vi "FPGA_DAC_move.vi"   [LabVIEW 2013]
uses:
  <vilib>/rvi/Emulation/niFpgaSctlEmulationGetInTimedLoop.vi
  <vilib>/rvi/Emulation/niFpgaEmulationReportErrorSimple.vi
  <vilib>/rvi/Emulation/niFpgaGetClockAttributes.vi
  <vilib>/rvi/FIFO/Fifo_Resource/nirvififoEmulationReadFpgaImpl.vi
  <vilib>/rvi/DataTransferAndStorage/Container/Common/niFpgaContainerGetUniqueNameForEmu.vi
  <vilib>/rvi/Emulation/niFpgaCriticalErrorInLSC.vi
  <vilib>/rvi/eio/common/nirviEmuTemplateMethod_errors.vi
  <vilib>/rvi/DataTransferAndStorage/Container/XNode/niFpgaContainer.xnode
  <vilib>/rvi/FIFO/Fifo_Resource/nirvififoEmulationRead.vi
  <vilib>/eio/EIONode/EIONode.xnode
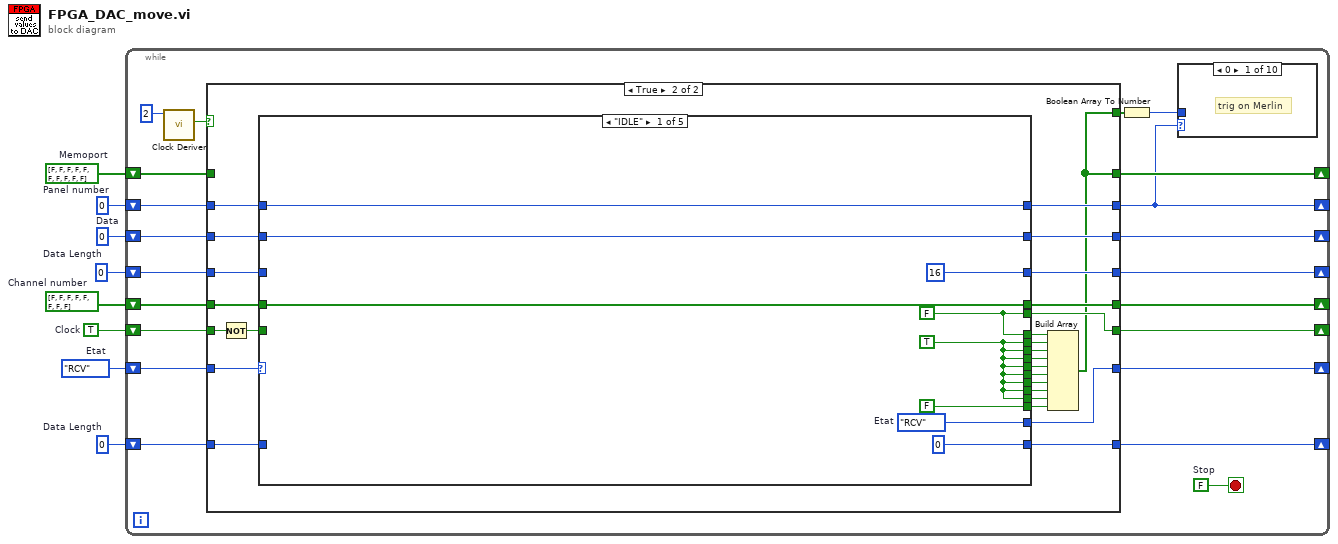
[diagram p0: block diagram]
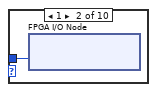
[diagram p2: hidden frame]
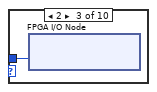
[diagram p3: hidden frame]
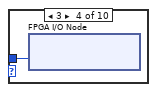
[diagram p4: hidden frame]
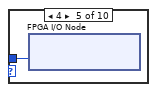
[diagram p5: hidden frame]
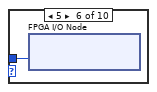
[diagram p6: hidden frame]
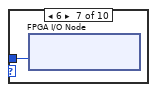
[diagram p7: hidden frame]
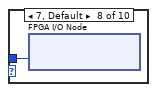
[diagram p8: hidden frame]
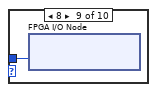
[diagram p9: hidden frame]
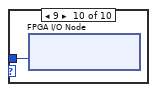
[diagram p10: hidden frame]
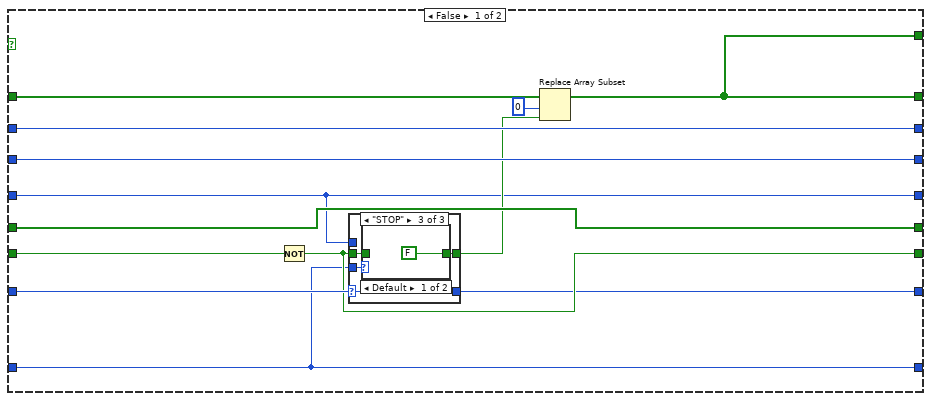
[diagram p11: hidden frame]
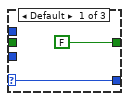
[diagram p12: hidden frame]
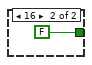
[diagram p14: hidden frame]
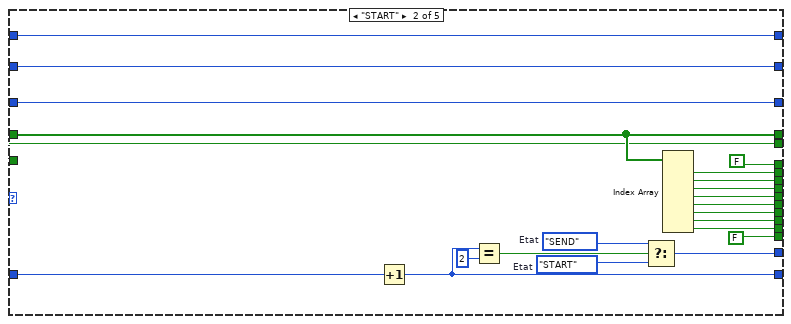
[diagram p16: hidden frame]
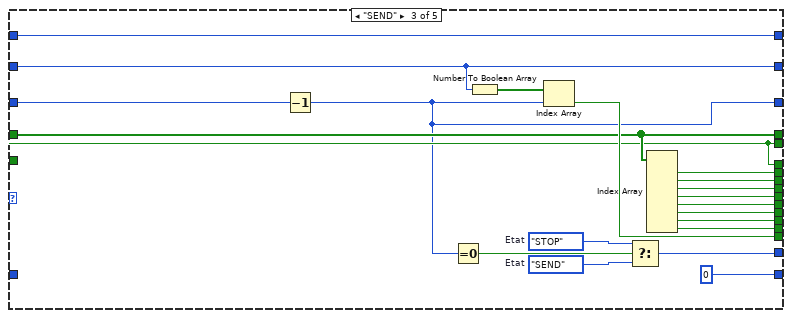
[diagram p17: hidden frame]
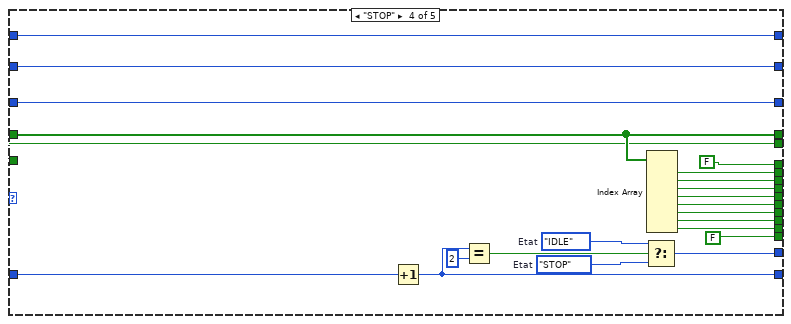
[diagram p18: hidden frame]
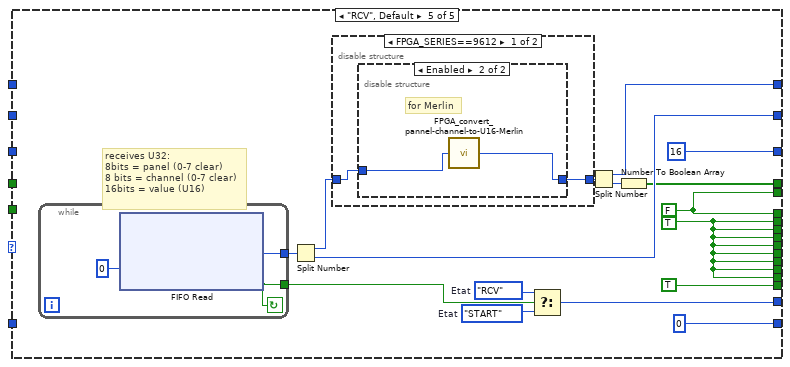
[diagram p19: hidden frame]
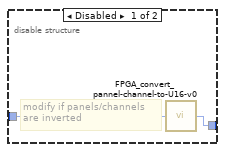
[diagram p20: hidden frame]
diagram:
  w1 = enum8{"IDLE", "START", "SEND", "STOP", "RCV"}."RCV"  # Etat
  w8 = u8 0  # Panel number
  w7 = bool[] [FALSE, FALSE, FALSE, FALSE, FALSE, FALSE, FALSE, FALSE]  # Channel number
  w6 = bool[] [FALSE, FALSE, FALSE, FALSE, FALSE, FALSE, FALSE, FALSE, FALSE, FALSE]  # Memoport
  w5 = u8 0  # Data Length
  w4 = 0  # Data Length
  w3 = u16 0  # Data
  w2 = TRUE  # Clock
  n1 = while {
    shift-right: [w23] -> _
    shift-left: w2 -> [w20]
    shift-right: [w29] -> _
    shift-left: w1 -> [w10]
    shift-right: [w28] -> _
    shift-left: w3 -> [w25]
    shift-right: [w27] -> _
    shift-left: w4 -> [w26]
    shift-right: [w22] -> _
    shift-left: w5 -> [w24]
    shift-right: [w19] -> _
    shift-left: w6 -> [w18]
    shift-right: [w17] -> _
    shift-left: w7 -> [w16]
    shift-right: [w13] -> _
    shift-left: w8 -> [w14]
    stop <- w9 stop-if-true
    w9 = FALSE  # Stop
    n2 = call "Clock Deriver.vi"("Divisor"=u32 2) -> ("Clock Out"=w21:bool)  [unwired: 1 in, 9 out]
    n3 = case shown="True" w21 {
      tunnel: w10 -> [w44 w91]
      tunnel: [w39 w90] -> w29
      tunnel: [w51 w89] -> w28
      tunnel: [w40 w88] -> w27
      tunnel: w26 -> [w40 w87]
      tunnel: w25 -> [w51 w86]
      tunnel: w20 -> [w47 w70]
      tunnel: w24 -> [w41 w85]
      tunnel: [w43 w69] -> w23
      tunnel: [w41 w84] -> w22
      tunnel: [w45 w67] -> w19
      tunnel: w18 -> [w50 _]
      tunnel: [w48 w75] -> w17
      tunnel: w16 -> [w48 w74]
      tunnel: [w46 w72] -> w13
      tunnel: w14 -> [w46 w73]
      tunnel: [w45 w67] -> w11
      frame False {
        n4 = Not(x=w47) -> (.not. x?=w43:bool)
        n5 = case shown="\"STOP\"" w44 {
          selector: w44 -> [w52 w54 w60]
          tunnel: w43 -> [_ w57 w62]
          tunnel: [FALSE w56 w61] -> w42
          tunnel: w41 -> [_ _ w63]
          tunnel: w40 -> [_ w55 _]
          tunnel: [w52 w54 w60] -> w39
          frame Default {
          }
          frame "SEND" {
            n6 = case shown="Default" w55 {
              tunnel: w57 -> [w58 _]
              tunnel: [w58 FALSE] -> w56
              frame Default {
              }
              frame 16 {
              }
            }
          }
          frame "STOP" {
            n7 = case shown="Default" w63 {
              tunnel: w62 -> [_ w65]
              tunnel: [FALSE w65] -> w61
              frame Default {
              }
              frame 0 {
              }
            }
          }
        }
        n8 = Replace Array Subset(array=w50, new element=w42, index=0) -> (w45:bool[])
      }
      frame True {
        n9 = Not(x=w70) -> (.not. x?=w68:bool)
        n10 = case shown="\"IDLE\"" w91 {
          tunnel: [w93 w118 w138 w161 w176] -> w90
          tunnel: [w98 w115 w135 w158 w181] -> w77
          tunnel: [w98 w114 w134 w157 w181] -> w78
          tunnel: [w98 w113 w133 w156 w181] -> w79
          tunnel: [w98 w111 w131 w154 w181] -> w81
          tunnel: [w98 w110 w130 w153 w181] -> w82
          tunnel: [w98 w109 w129 w152 w181] -> w83
          tunnel: [FALSE ("CS") FALSE ("CS") w142 FALSE ("CS") TRUE ("CS")] -> w71
          tunnel: [w98 w112 w132 w155 w181] -> w80
          tunnel: [w94 w122 w140 w164 w178] -> w89
          tunnel: [16 ("Data Length") w121 w125 w163 16 ("Data Length")] -> w88
          tunnel: w87 -> [_ w121 w141 w163 _]
          tunnel: w86 -> [w94 w122 w140 w164 _]
          tunnel: w68 -> [_ w106 w126 w149 _]
          tunnel: w85 -> [_ w117 _ w162 _]
          tunnel: [w92 w106 w126 w149 w166] -> w69
          tunnel: [u8 0 ("Data Length") w102 u8 0 ("Data Length") w145 u8 0 ("Data Length")] -> w84
          tunnel: [w98 w116 w136 w159 w181] -> w76
          tunnel: [w96 w108 w128 w151 w177] -> w75
          tunnel: w74 -> [w96 w108 w128 w151 _]
          tunnel: [w95 w107 w127 w150 w168] -> w72
          tunnel: w73 -> [w95 w107 w127 w150 _]
          tunnel: [w92 FALSE w126 FALSE w166] -> w66
          frame "IDLE" {
            w93 = enum8{"IDLE", "START", "SEND", "STOP", "RCV"}."RCV"  # Etat
            w92 = FALSE
            w98 = TRUE ("CS")
          }
          frame "START" {
            w103 = enum8{"IDLE", "START", "SEND", "STOP", "RCV"}."START"  # Etat
            w104 = enum8{"IDLE", "START", "SEND", "STOP", "RCV"}."SEND"  # Etat
            n11 = Increment(x=w117) -> (x+1=w102:u8)
            n12 = Equal?(x=w102, y=u8 2) -> (x = y?=w119:bool)
            n13 = Select(t=w104, s=w119, f=w103) -> (s? t:f=w118:enum8{"IDLE", "START", "SEND", "STOP", "RCV"})
            n14 = Index Array(array=w108) -> (element #1=w116:bool, element #2=w115:bool, element #3=w114:bool, element #4=w113:bool, element #5=w112:bool, element #6=w111:bool, element #7=w110:bool, element #8=w109:bool)  [unwired: 8 in]
          }
          frame "SEND" {
            w123 = enum8{"IDLE", "START", "SEND", "STOP", "RCV"}."SEND"  # Etat
            w124 = enum8{"IDLE", "START", "SEND", "STOP", "RCV"}."STOP"  # Etat
            n15 = Decrement(x=w141) -> (x-1=w125:i32)
            n16 = Equal To 0?(x=w125) -> (x = 0?=w139:bool)
            n17 = Number To Boolean Array(number=w140) -> (Boolean array=w143:bool[])
            n18 = Index Array(array=w143, index=w125) -> (element=w142:bool)
            n19 = Select(t=w124, s=w139, f=w123) -> (s? t:f=w138:enum8{"IDLE", "START", "SEND", "STOP", "RCV"})
            n20 = Index Array(array=w128) -> (element #1=w136:bool, element #2=w135:bool, element #3=w134:bool, element #4=w133:bool, element #5=w132:bool, element #6=w131:bool, element #7=w130:bool, element #8=w129:bool)  [unwired: 8 in]
          }
          frame "STOP" {
            w146 = enum8{"IDLE", "START", "SEND", "STOP", "RCV"}."STOP"  # Etat
            w147 = enum8{"IDLE", "START", "SEND", "STOP", "RCV"}."IDLE"  # Etat
            n21 = Increment(x=w162) -> (x+1=w145:u8)
            n22 = Equal?(x=w145, y=u8 2) -> (x = y?=w160:bool)
            n23 = Select(t=w147, s=w160, f=w146) -> (s? t:f=w161:enum8{"IDLE", "START", "SEND", "STOP", "RCV"})
            n24 = Index Array(array=w151) -> (element #1=w159:bool, element #2=w158:bool, element #3=w157:bool, element #4=w156:bool, element #5=w155:bool, element #6=w154:bool, element #7=w153:bool, element #8=w152:bool)  [unwired: 8 in]
          }
          frame "RCV", Default {
            w171 = enum8{"IDLE", "START", "SEND", "STOP", "RCV"}."RCV"  # Etat
            w172 = enum8{"IDLE", "START", "SEND", "STOP", "RCV"}."START"  # Etat
            w166 = FALSE
            w181 = TRUE ("CS")
            # "receives U32:\n8bits = panel (0-7 clear)\n8 bits = channel (0-7 clear)\n16bits = value (U16)"
            n25 = while {
              tunnel: [w184] -> w174
              tunnel: [w182] -> w173
              stop <- w182 continue-if-true
              n26 = xnode ("FIFO Read")("Timeout"=0) -> ("Element"=w184:u32, "Timed Out?"=w182:bool)  [unwired: 1 in, 1 out]
            }
            n27 = Split Number(x=w174) -> (hi(x)=w170:u16, lo(x)=w178:u16)
            n28 = disable-structure shown="FPGA_SERIES==9612" {
              disable-tunnel: [w186 w191] -> w169
              disable-tunnel: w170 -> [w185 w192]
              frame condition #0 (active) {
                n29 = disable-structure shown="Enabled" {
                  disable-tunnel: [w188 w190] -> w186
                  disable-tunnel: w185 -> [w187 w189]
                  frame Disabled {
                    # "modify if panels/channels\nare inverted"
                    n30 = call "FPGA_convert_pannel-channel-to-U16-v0.vi"("pannel|channel"=w187) -> ("Numérique"=w188:u16)
                  }
                  frame Enabled {
                    # "for Merlin"
                    n31 = call "FPGA_convert_pannel-channel-to-U16-Merlin.vi"("pannel|channel"=w189) -> ("Numérique"=w190:u16)
                  }
                }
              }
              frame condition #1 {
                n32 = call "FPGA_convert_pannel-channel-to-U16-v1.vi"("pannel|channel"=w192) -> ("Numérique"=w191:u16)
              }
            }
            n33 = Select(t=w171, s=w173, f=w172) -> (s? t:f=w176:enum8{"IDLE", "START", "SEND", "STOP", "RCV"})
            n34 = Split Number(x=w169) -> (hi(x)=w168:u8, lo(x)=w167:u8)
            n35 = Number To Boolean Array(number=w167) -> (Boolean array=w177:bool[])
          }
        }
        n36 = Build Array(w66, w76, w77, w78, w79, w80, w81, w82, w83, w71) -> (w67:bool[])
      }
    }
    n37 = Boolean Array To Number(Boolean array=w11) -> (number=w12:u16)
    n38 = case shown="0" w13 {
      tunnel: w12 -> [_ w30 w31 w32 w33 w34 w35 w36 w37 w38]
      frame 0 {
        # "trig on Merlin"
      }
      frame 1 {
        n39 = xnode "FPGA I/O Node"("Port1/DIO9:0"=w30) -> ()  [unwired: 1 in, 1 out]
      }
      frame 2 {
        n40 = xnode "FPGA I/O Node"("Port2/DIO9:0"=w31) -> ()  [unwired: 1 in, 1 out]
      }
      frame 3 {
        n41 = xnode "FPGA I/O Node"("Port3/DIO9:0"=w32) -> ()  [unwired: 1 in, 1 out]
      }
      frame 4 {
        n42 = xnode "FPGA I/O Node"("Port4/DIO9:0"=w33) -> ()  [unwired: 1 in, 1 out]
      }
      frame 5 {
        n43 = xnode "FPGA I/O Node"("Port5/DIO9:0"=w34) -> ()  [unwired: 1 in, 1 out]
      }
      frame 6 {
        n44 = xnode "FPGA I/O Node"("Port6/DIO9:0"=w35) -> ()  [unwired: 1 in, 1 out]
      }
      frame 7, Default {
        n45 = xnode "FPGA I/O Node"("Port7/DIO9:0"=w36) -> ()  [unwired: 1 in, 1 out]
      }
      frame 8 {
        n46 = xnode "FPGA I/O Node"("Port8/DIO9:0"=w37) -> ()  [unwired: 1 in, 1 out]
      }
      frame 9 {
        n47 = xnode "FPGA I/O Node"("Port9/DIO9:0"=w38) -> ()  [unwired: 1 in, 1 out]
      }
    }
  }
